vi "set_parameters.vi"(8 "error in (no error)":errorcluster) -> (0 "error out (no error)":errorcluster)   [LabVIEW 2019, in "Glaz.lvclass"]
uses:
  Glaz.lvclass
panel:
  in  "script file":path
  in  "continue":bool
  in  "Integration\nTime [us]":i32=2
  in  "HW Averaging":T1(ring)
  in  "Trigger Mode":enum16{"External", "Internal", "Burst"}(ring)=enum."Internal"
  in  "Integration Mode":enum16{"PulseSync", "TimeFill"}(ring)
  in  "scanCount":i32=500
  in  "trig delay":i32
  in  "internal freq":dbl=3000.0
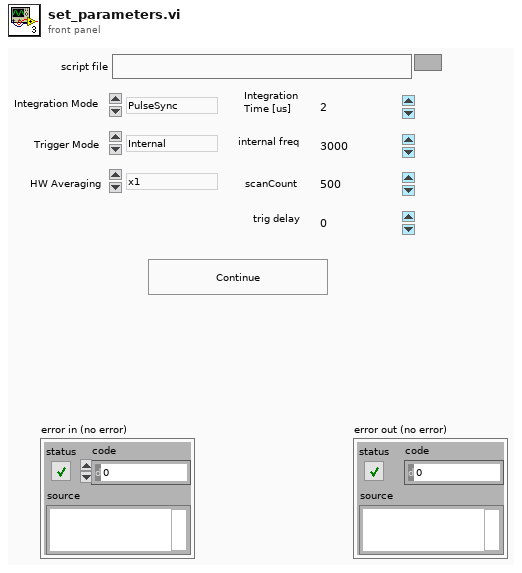
[diagram p1: front panel]
types:
  T1 = enum16{"x1", "x2", "x4", "x8", "x16", "x32", "x64", "x128", "x256"}
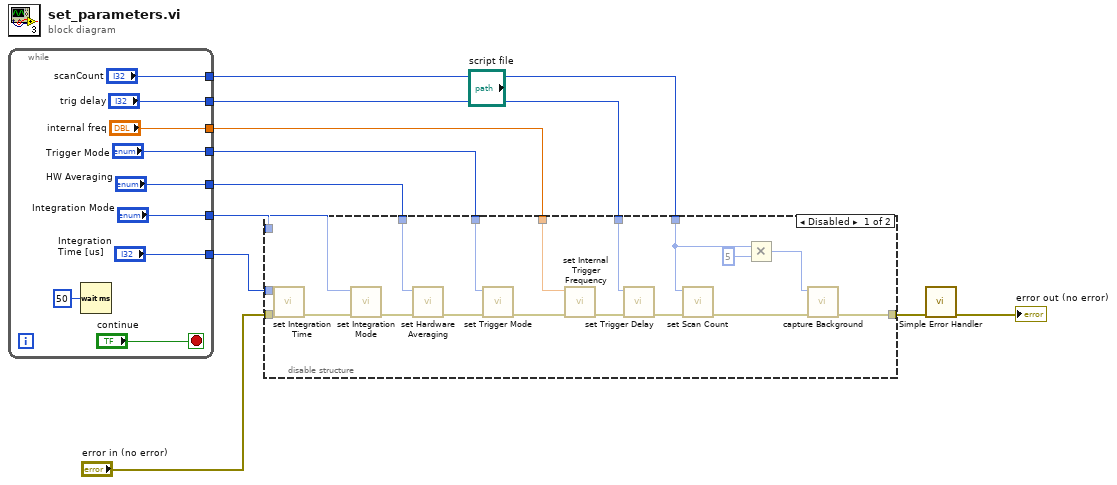
[diagram p0: block diagram]
diagram:
  n1 = while {
    tunnel: ["internal freq"] -> w9
    tunnel: ["trig delay"] -> w8
    tunnel: ["Integration Mode"] -> w7
    tunnel: ["Trigger Mode"] -> w6
    tunnel: ["HW Averaging"] -> w5
    tunnel: ["Integration\nTime [us]"] -> w4
    tunnel: ["scanCount"] -> w3
    stop <- "continue" stop-if-true
    n2 = Wait (ms)(milliseconds to wait=u32 50) -> ()  [unwired: 1 out]
  }
  n3 = disable-structure shown="Disabled" {
    disable-tunnel: "error in (no error)" -> [w31 _]
    disable-tunnel: w9 -> [w30 _]
    disable-tunnel: w8 -> [w29 _]
    disable-tunnel: w7 -> [w28 _]
    disable-tunnel: w6 -> [w27 _]
    disable-tunnel: w5 -> [w26 _]
    disable-tunnel: w4 -> [w25 _]
    disable-tunnel: w3 -> [w23 _]
    disable-tunnel: [w20 _] -> w2
    frame Disabled {
      n4 = call <userlib>:"set Integration Time.vi"("error in (no error)"=w31, "us"=w25) -> ("error out"=w32:errorcluster)  [unwired: 8 in, 1 out]
      n5 = call <userlib>:"set Integration Mode.vi"("error in (no error)"=w32, "mode"=w28) -> ("error out"=w33:errorcluster)  [unwired: 8 in, 1 out]
      n6 = call <userlib>:"set Hardware Averaging.vi"("error in (no error)"=w33, "averaging"=w26) -> ("error out"=w34:errorcluster)  [unwired: 8 in, 1 out]
      n7 = call <userlib>:"set Trigger Mode.vi"("error in (no error)"=w34, "mode"=w27) -> ("error out"=w35:errorcluster)  [unwired: 8 in, 1 out]
      n8 = call <userlib>:"set Internal Trigger Frequency.vi"("error in (no error)"=w35, "Hz"=w30) -> ("error out"=w36:errorcluster)  [unwired: 8 in, 1 out]
      n9 = call <userlib>:"set Trigger Delay.vi"("error in (no error)"=w36, "us"=w29) -> ("error out"=w37:errorcluster)  [unwired: 8 in, 1 out]
      n10 = call <userlib>:"set Scan Count.vi"("error in (no error)"=w37, "scanCount"=w23) -> ("error out"=w24:errorcluster)  [unwired: 8 in, 1 out]
      n11 = Multiply(x=w23, y=5) -> (x*y=w21:i32)
      n12 = call <userlib>:"capture Background.vi"("error in (no error)"=w24, "scanCount"=w21) -> ("error out"=w20:errorcluster)  [unwired: 8 in, 1 out]
    }
    frame Enabled {
    }
  }
  n13 = call <vilib>:"Simple Error Handler.vi"("error in (no error)"=w2) -> ("error out"=→"error out (no error)":errorcluster)  [unwired: 4 in, 4 out]
